vi "ACK.vi"(11 "Python in":string="import machine, utime\n\ntx = machine.Pin('Y9', machine.Pin.OUT)\nrx = machine.Pin('Y10', machine.Pin.IN)\ntx.value(b'\\x00')\nutime.sleep_ms(500)\ntx.value(1)\n\nuart = machine.UART(3)\nuart.init(baudrate=2400, bits=8, parity=None, stop=1)\n\nuart.write(0)\nuart.write(b'\\x40\\x23\\x9C')\nuart.write(b'\\x98\\x00\\x4C\\x69\\x67\\x68\\x74\\x00\\x00\\x00\\x39')\nuart.write(b'\\x90\\x80\\x01\\x00\\x03\\x00\\xED')\n") -> (3 "Python out":string="import machine, utime\n\ntx = machine.Pin('Y9', machine.Pin.OUT)\nrx = machine.Pin('Y10', machine.Pin.IN)\ntx.value(b'\\x00')\nutime.sleep_ms(500)\ntx.value(1)\n\nuart = machine.UART(3)\nuart.init(baudrate=2400, bits=8, parity=None, stop=1)\n\nuart.write(0)\nuart.write(b'\\x40\\x23\\x9C')\nuart.write(b'\\x98\\x00\\x4C\\x69\\x67\\x68\\x74\\x00\\x00\\x00\\x39')\nuart.write(b'\\x90\\x80\\x01\\x00\\x03\\x00\\xED')\nuart.write(b'\\x04')\n")   [LabVIEW 2016]
panel:
  out "bytes added":u8[](array[numeric])=[4]
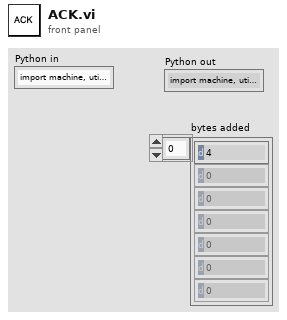
[diagram p1: front panel]
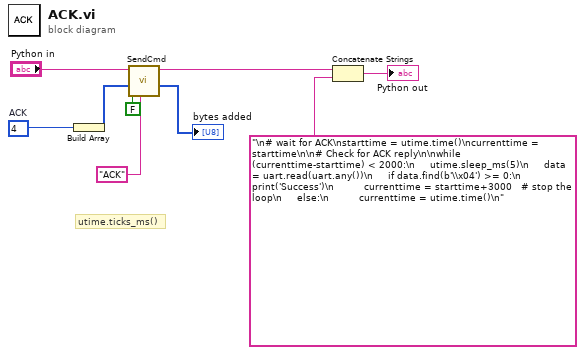
[diagram p0: block diagram]
diagram:
  w6 = u8 4  # ACK
  # "utime.ticks_ms()"
  n1 = Build Array(w6) -> (w7:u8[])
  n2 = call "SendCmd.vi"("Comment"="ACK", "Add Chksm"=FALSE, "Array In"=w7, "Python in"="Python in") -> ("Array Sent"=→"bytes added":u8[], "Python out"=w3:string)  [unwired: 6 in]
  n3 = Concatenate Strings(w3, "\n# wait for ACK\nstarttime = utime.time()\ncurrenttime = starttime\n\n# Check for ACK reply\n\nwhile (currenttime-starttime) < 2000:\n     utime.sleep_ms(5)\n     data = uart.read(uart.any())\n     if data.find(b'\\x04') >= 0:\n          print('Success')\n          currenttime = starttime+3000   # stop the loop\n     else:\n          currenttime = utime.time()\n" ("Python in")) -> (→"Python out":string)
